vi "Demo.vi"() -> ()   [LabVIEW 2021, in "TipStripOOPanelExample.lvlib"]
uses:
  TipStripOOPanelExample.lvlib
  TipPanelExampleClass/TipPanelExample.lvclass
  C:/GIT checkouts/TipStrip-OOPanel/Source/Classes/TipPanel/TipPanel.lvclass
  Classes/TipPanelHandle/CMD - shutdown.vi
  Classes/TipPanelHandle/CMD - show panel.vi
  Classes/TipPanelHandle/CMD - hide.vi
  Classes/TipPanelHandle/TipPanelHandle.lvclass
  C:/Program Files/National Instruments/LabVIEW 2021/vi.lib/IlluminatedG/IG OOPanel/OOPanel/Panel/Panel.lvclass
  C:/GIT checkouts/TipStrip-OOPanel/Source/Example/TipPanelExampleClass/TipPanelExample.lvclass
panel:
  out "Table Control":string[][](table)
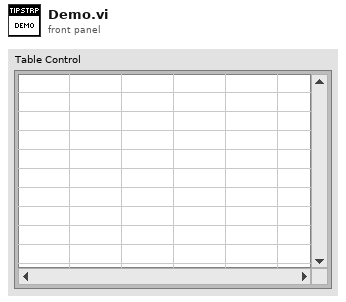
[diagram p1: front panel]
types:
  T1 = typedef "LVPoint32TypeDef.ctl" = cluster{"Horizontal":i32, "Vertical":i32}
  T2 = typedef "LVRowAndColumnTypeDef.ctl" = cluster{"Row":i32, "Column":i32}
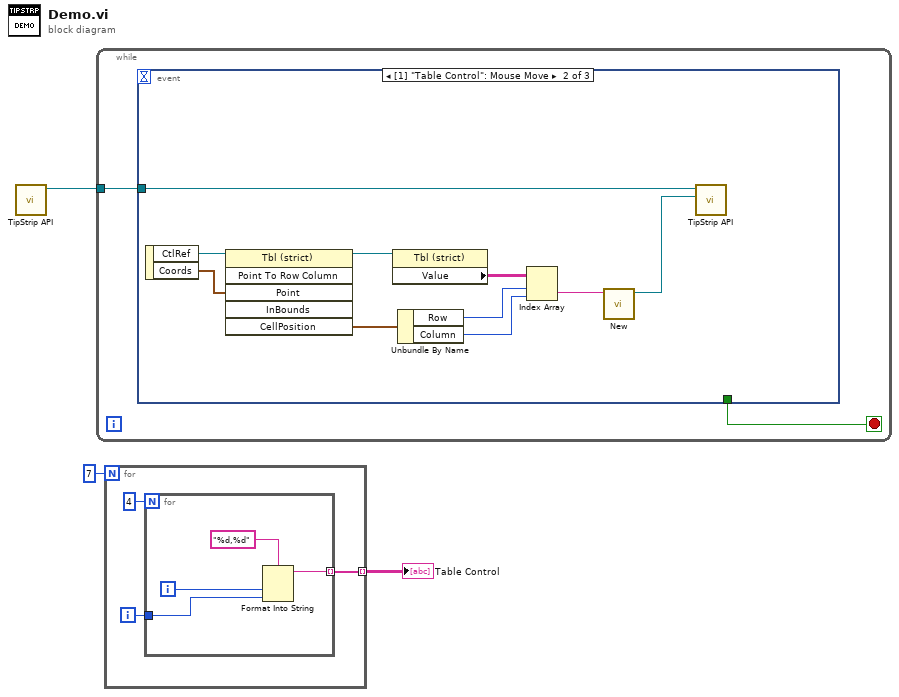
[diagram p0: block diagram]
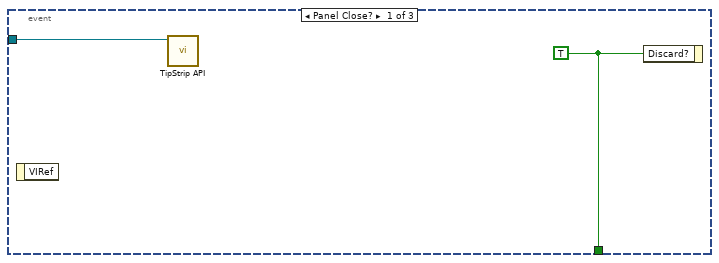
[diagram p2: hidden frame]
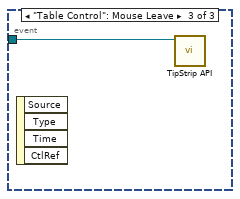
[diagram p3: hidden frame]
diagram:
  n1 = call-poly "TipStrip API.vi"() -> ("TipPanelHandle out"=w3:refnum<class "TipPanelHandle.lvclass">)  [unwired: 10 in, 1 out]
  n2 = while {
    tunnel: w3 -> [w4]
    stop <- w5 stop-if-true
    n3 = event shown="[1] \"Table Control\": Mouse Move" {
      selector: _ -> [_ _ _]
      dyn-events: _ -> [_ _ _]
      timeout: _ -> [_ _ _]
      tunnel: [w7 _ _] -> w5
      tunnel: w4 -> [w6 w10 w18]
      event Panel Close? {
        w7 = TRUE ("Discard?")
        n4 = event-data() -> ()  [unwired: 1 in, 1 out]
        n5 = call-poly "TipStrip API.vi"("TipPanelHandle"=w6) -> ()  [unwired: 10 in, 1 out]
        n6 = event-data("Discard?"=w7) -> ()  [unwired: 1 in, 1 out]
      }
      event "Table Control": Mouse Move {
        n7 = event-data() -> ("CtlRef"=w17:refnum<vi>, "Coords"=w16:T1)  [unwired: 1 in]
        n8 = invoke class="Tbl (strict)" method="Point To Row Column"(reference=w17, "Point"=w16) -> (reference out=w15:refnum<vi>, "CellPosition"=w13:T2)  [unwired: 4 in, 4 out]
        n9 = property class="Tbl (strict)"(reference=w15) -> ("Value"=w14:string[][])  [unwired: 1 in, 2 out]
        n10 = Unbundle By Name(w13) -> ("Row"=w12:i32, "Column"=w11:i32)
        n11 = Index Array(array=w14, index (row)=w12, index (col)=w11) -> (element=w9:string)
        n12 = call "New.vi"("MyData"=w9) -> ("TipPanelExample out"=w8:refnum<class "TipPanelExample.lvclass">)  [unwired: 9 in, 1 out]
        n13 = call-poly "TipStrip API.vi"("TipPanel"=w8, "TipPanelHandle"=w10) -> ()  [unwired: 8 in, 2 out]
      }
      event "Table Control": Mouse Leave {
        n14 = event-data() -> ()  [unwired: 1 in, 4 out]
        n15 = call-poly "TipStrip API.vi"("TipPanelHandle"=w18) -> ()  [unwired: 9 in, 2 out]
      }
    }
  }
  n16 = for {
    N: 7 -> [_]
    tunnel: [w20] -> w2 mode=indexing
    i -> [w21]
    n17 = for {
      N: 4 -> [_]
      tunnel: w21 -> [w23]
      tunnel: [w22] -> w20 mode=indexing
      i -> [w24]
      n18 = Format Into String(format string="%d,%d", w24, w23) -> (resulting string=w22:string)  [unwired: 2 in, 1 out]
    }
  }
  "Table Control" <- w2
